vi "ui_Library Query Listed String.vi"(0 "prompt":string, 7 "list of strings":string[](array[string]), 11 "default (persist)":string) -> (4 "OKed?":bool, 8 "selected string":string)   [LabVIEW 2012]
doc: "Allows a string to be easily selected from a list of candidate strings. The prompt explaining what is in need of being selected is shown in the titlebar. It is possible to type in the string, pick it from the list, or type part of the string until the list of candidates is sufficiently reduced to allow quick selection from the list."
uses:
  typedefs/t_Library Query Listed String States.ctl
panel:
  in  "selected":string
  in  "list":i32(listbox)
  in  "cancel":bool
  in  "OK":bool
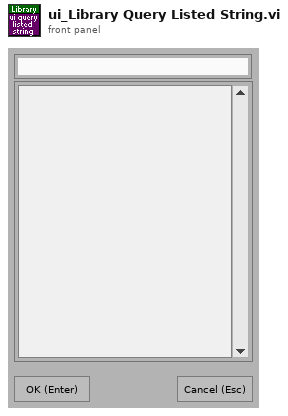
[diagram p1: front panel]
types:
  T1 = typedef "t_Library Query Listed String States.ctl" = enum16{"empty queue", "poll size", "update selected", "filter list", "show list", "OK", "initialize", "init controls", "init check list", "init persist", "init filter", "cleanup", "stop"}
  T2 = typedef "lveventtype.ctl" = enum32{"Null", "Timeout", "Annotation Menu Selection", "Annotation Menu Selection?", "App Instance Close", "App Instance Close?", "Autoscale Range Change", "Cell Edit", "Cell Edit?", "Cursor Grab", "Cursor Grab?", "Cursor Menu Selection", "Cursor Menu Selection?", "Cursor Move", "Cursor Release", "Data Change", "Direction Change", "Display State Change", "Drag Ended", "Drag Enter", "Drag Leave", "Drag Over", "Drag Source Update", "Drag Starting", "Drag Starting?", "Drop", "Exec State Change", "Key Down", "Key Down?", "Key Repeat", "Key Repeat?", "Key Up", "Listbox Double Click", "Menu Activation?", "Menu Selection (App)", "Menu Selection? (App)", "Menu Selection (User)", "Mouse Down", "Mouse Down?", "Mouse Enter", "Mouse Leave", "Mouse Move", "Mouse Up", "NI Security User Change (App)", "Pane Size", "Panel Close", "Panel Close?", "Panel Resize", "Plot Attribute Change", "Scale Range Change", "Shortcut Menu Activation?", "Shortcut Menu Selection (App)", "Shortcut Menu Selection? (App)", "Shortcut Menu Selection (User)", "Tree Double Click", "Tree Drag", "Tree Drag?", "Tree Drop", "Tree Drop?", "Tree Item Close", "Tree Item Close?", "Tree Item Open", "Tree Item Open?", "Value Change"}
  T3 = typedef "eventvkey.ctl" = enum16{"ASCII", "Enter", "Return", "Shift", "Ctrl", "Alt", "Cmd", "Opt", "Caps", "NumLock", "Clear", "Break", "Up", "Down", "Left", "Right", "Insert", "Delete", "Home", "End", "PageUp", "PageDown", "Escape", "Help", "Pause", "ScrollLock", "F1", "F2", "F3", "F4", "F5", "F6", "F7", "F8", "F9", "F10", "F11", "F12", "F13", "F14", "F15", "F16", "F17", "F18", "F19", "F20", "F21", "F22", "F23", "F24", "Play", "VolumeUp", "VolumeDown", "Mute", "Two Byte Char"}
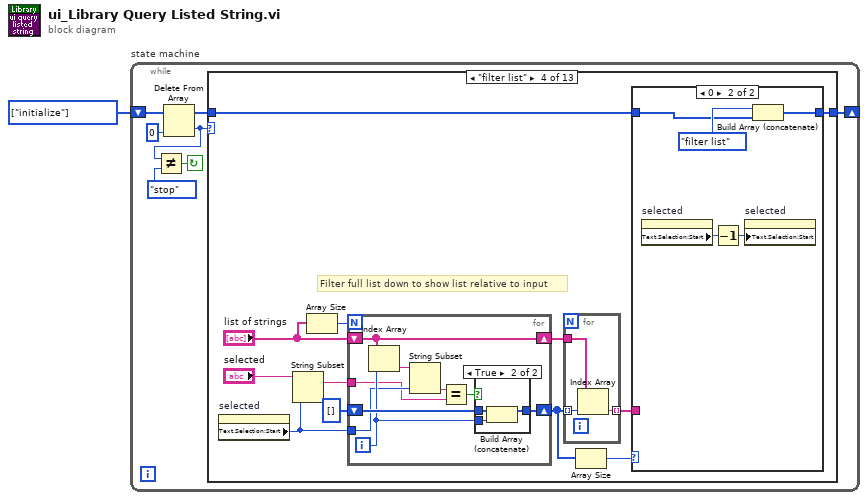
[diagram p0: block diagram]
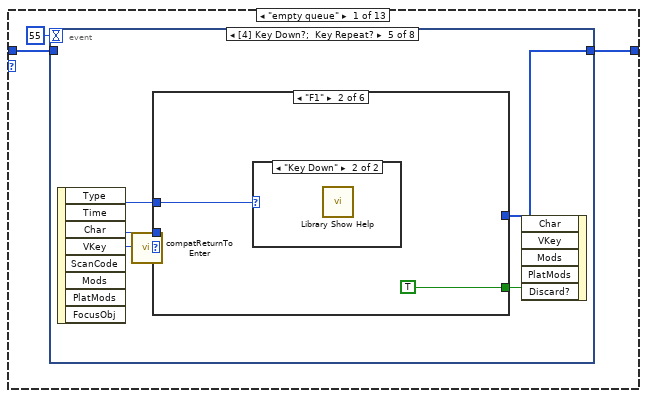
[diagram p2: hidden frame]
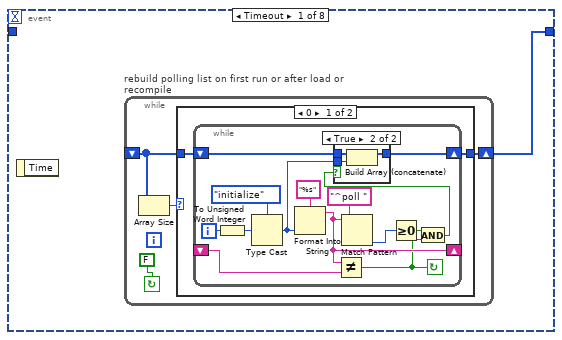
[diagram p3: hidden frame]
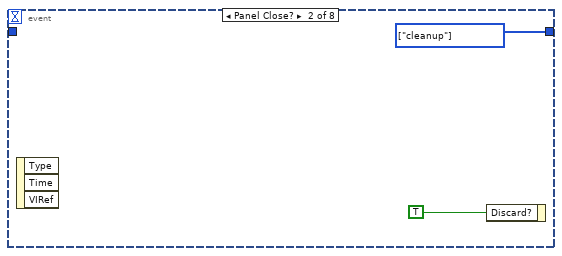
[diagram p6: hidden frame]
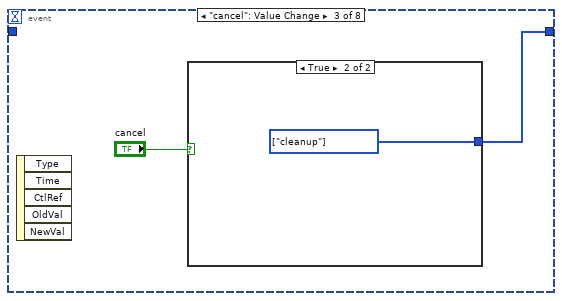
[diagram p7: hidden frame]
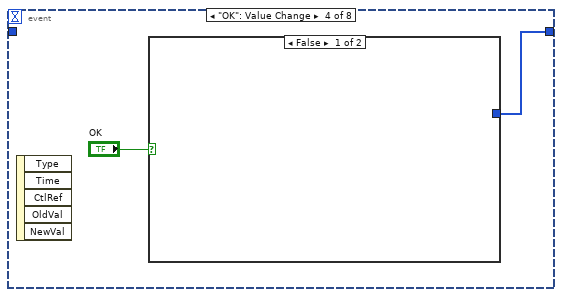
[diagram p9: hidden frame]
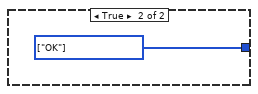
[diagram p10: hidden frame]
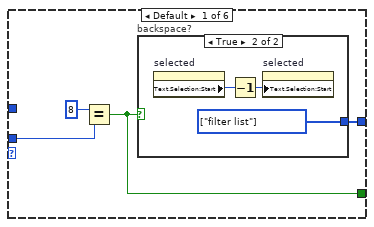
[diagram p11: hidden frame]
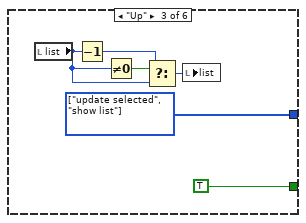
[diagram p14: hidden frame]
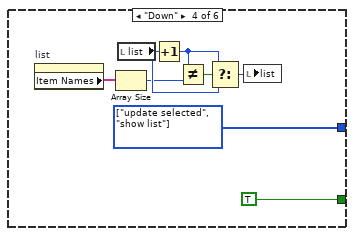
[diagram p15: hidden frame]
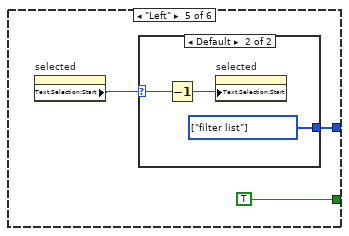
[diagram p16: hidden frame]
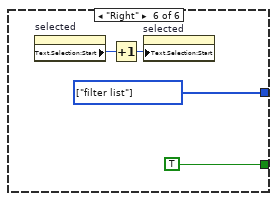
[diagram p18: hidden frame]
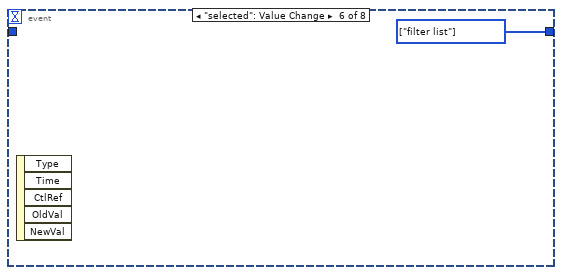
[diagram p19: hidden frame]
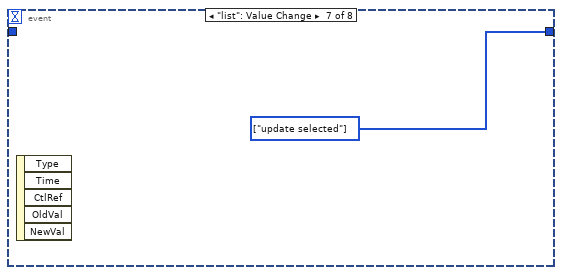
[diagram p20: hidden frame]
diagram:
  w1 = T1[] [enum."initialize"] items=["empty queue", "poll size", "update selected", "filter list", "show list", "OK", "initialize", "init controls", "init check list", "init persist", "init filter", "cleanup", "stop"] ("Array Constant")
  n1 = while "state machine" {
    shift-left: w1 -> [w5]
    shift-right: [w8] -> _
    stop <- w7 continue-if-true
    n2 = Delete From Array(array=w5, index=0) -> (deleted portion=w2:T1, array with subset deleted=w4:T1[])  [unwired: 1 in]
    n3 = Not Equal?(x=w2, y=t_Library_Query_Listed_String_States."stop" ("states")) -> (x != y?=w7:bool)
    n4 = case "Case" shown="\"filter list\"" w2 {
      tunnel: [w11 w91 w108 w119 w146 w180 w182 w212 w214 w220 w230 w234 w235] -> w8
      tunnel: w4 -> [w9 w91 w108 w120 w146 _ _ w212 w215 w220 w231 _ w235]
      frame "empty queue" {
        n5 = event shown="[4] Key Down?;  Key Repeat?" {
          selector: _ -> [_ _ _ _ _ _ _ _]
          dyn-events: _ -> [_ _ _ _ _ _ _ _]
          timeout: 55 -> [_ _ _ _ _ _ _ _]
          tunnel: [w12 w39 w40 w43 w48 w85 w86 w88] -> w11
          tunnel: w9 -> [_ _ _ _ _ _ _ _]
          event Timeout {
            n6 = event-data() -> ()  [unwired: 1 in, 1 out]
            n7 = while "rebuild polling list on first run or after load or recompile" {
              shift-left: _ -> [w15]
              shift-right: [w14] -> w12
              stop <- FALSE continue-if-true
              n8 = Array Size(array=w15) -> (size(s)=w16:i32)
              n9 = case shown="0" w16 {
                tunnel: [w17 w37] -> w14
                tunnel: w15 -> [w18 w37]
                frame 0 {
                  n10 = while {
                    shift-left: w18 -> [w27]
                    shift-right: [w25] -> w17
                    shift-left: _ -> [w29]
                    shift-right: [w24] -> _
                    i -> [w32]
                    stop <- w20 continue-if-true
                    n11 = To Unsigned Word Integer(number=w32) -> (unsigned 16bit integer=w30:u16)
                    n12 = Type Cast(type=t_Library_Query_Listed_String_States."initialize" ("states"), x=w30) -> (*(type *) &x=w26:T1)
                    n13 = Format Into String(format string="%s" ("Format String"), w26) -> (resulting string=w24:string)  [unwired: 2 in, 1 out]
                    n14 = Not Equal?(x=w24, y=w29) -> (x != y?=w20:bool)
                    n15 = Match Pattern(string=w24, regular expression="^poll ") -> (offset past match=w22:i32)  [unwired: 1 in, 3 out]
                    n16 = Greater Or Equal To 0?(x=w22) -> (x >= 0?=w21:bool)
                    n17 = And(x=w21, y=w20) -> (x .and. y?=w19:bool)
                    n18 = case shown="True" w19 {
                      tunnel: w27 -> [w33 w36]
                      tunnel: w26 -> [_ w35]
                      tunnel: [w33 w34] -> w25
                      frame False {
                      }
                      frame True {
                        n19 = Build Array (concatenate)(w36, w35) -> (w34:T1[])
                      }
                    }
                  }
                }
                frame Default {
                }
              }
            }
          }
          event Panel Close? {
            w39 = T1[] [enum."cleanup"] items=["empty queue", "poll size", "update selected", "filter list", "show list", "OK", "initialize", "init controls", "init check list", "init persist", "init filter", "cleanup", "stop"] ("Array Constant")
            n20 = event-data() -> ()  [unwired: 1 in, 3 out]
            n21 = event-data("Discard?"=TRUE) -> ()  [unwired: 1 in, 1 out]
          }
          event "cancel": Value Change {
            n22 = event-data() -> ()  [unwired: 1 in, 5 out]
            n23 = case shown="True" "cancel" {
              tunnel: [_ w42] -> w40
              frame False {
              }
              frame True {
                w42 = T1[] [enum."cleanup"] items=["empty queue", "poll size", "update selected", "filter list", "show list", "OK", "initialize", "init controls", "init check list", "init persist", "init filter", "cleanup", "stop"] ("Array Constant")
              }
            }
          }
          event "OK": Value Change {
            n24 = event-data() -> ()  [unwired: 1 in, 5 out]
            n25 = case shown="False" "OK" {
              tunnel: [_ w45] -> w43
              frame False {
              }
              frame True {
                w45 = T1[] [enum."OK"] items=["empty queue", "poll size", "update selected", "filter list", "show list", "OK", "initialize", "init controls", "init check list", "init persist", "init filter", "cleanup", "stop"] ("Array Constant")
              }
            }
          }
          event Key Down?; event type 5.0.x8000000b {
            n26 = event-data() -> ("Type"=w47:T2, "Char"=w49:i16, "VKey"=w46:T3)  [unwired: 1 in, 5 out]
            n27 = call <vilib>:"compatReturnToEnter.vi"("VKey"=w46) -> ("VKey"=w51:T3)
            n28 = case shown="\"F1\"" w51 {
              tunnel: [w52 TRUE ("Discard?") TRUE ("Discard?") TRUE ("Discard?") TRUE ("Discard?") TRUE ("Discard?")] -> w50
              tunnel: w49 -> [w55 _ _ _ _ _]
              tunnel: [w53 _ w66 w74 w76 w83] -> w48
              tunnel: w47 -> [_ w59 _ _ _ _]
              frame Default {
                n29 = Equal?(x=i16 8, y=w55) -> (x = y?=w52:bool)
                n30 = case "backspace?" shown="True" w52 {
                  tunnel: [_ w58] -> w53
                  frame False {
                  }
                  frame True {
                    w58 = T1[] [enum."filter list"] items=["empty queue", "poll size", "update selected", "filter list", "show list", "OK", "initialize", "init controls", "init check list", "init persist", "init filter", "cleanup", "stop"] ("Array Constant")
                    n31 = property on="selected" class="Str"() -> ("Text.Selection:Start"=w57:u32)  [unwired: 2 in, 2 out]
                    n32 = Decrement(x=w57) -> (x-1=w56:u32)
                    n33 = property on="selected" class="Str"("Text.Selection:Start"=w56) -> ()  [unwired: 2 in, 2 out]
                  }
                }
              }
              frame "F1" {
                n34 = case shown="\"Key Down\"" w59 {
                  frame Default {
                  }
                  frame "Key Down" {
                    n35 = call "Library Show Help.vi"() -> ()  [unwired: 1 in]
                  }
                }
              }
              frame "Up" {
                w66 = T1[] [enum."update selected", enum."show list"] items=["empty queue", "poll size", "update selected", "filter list", "show list", "OK", "initialize", "init controls", "init check list", "init persist", "init filter", "cleanup", "stop"] ("Array Constant")
                n36 = local read "list"() -> (w61:i32)
                n37 = Decrement(x=w61) -> (x-1=w62:i32)
                n38 = Not Equal To 0?(x=w61) -> (x != 0?=w64:bool)
                n39 = Select(t=w62, s=w64, f=w61) -> (s? t:f=w63:i32)
                n40 = local write "list"(w63) -> ()
              }
              frame "Down" {
                w74 = T1[] [enum."update selected", enum."show list"] items=["empty queue", "poll size", "update selected", "filter list", "show list", "OK", "initialize", "init controls", "init check list", "init persist", "init filter", "cleanup", "stop"] ("Array Constant")
                n41 = property on="list" class="LstBox (strict)"() -> ("Item Names"=w67:string[])  [unwired: 2 in, 2 out]
                n42 = Array Size(array=w67) -> (size(s)=w68:i32)
                n43 = local read "list"() -> (w69:i32)
                n44 = Increment(x=w69) -> (x+1=w70:i32)
                n45 = Not Equal?(x=w70, y=w68) -> (x != y?=w72:bool)
                n46 = Select(t=w70, s=w72, f=w69) -> (s? t:f=w71:i32)
                n47 = local write "list"(w71) -> ()
              }
              frame "Left" {
                n48 = property on="selected" class="Str"() -> ("Text.Selection:Start"=w75:u32)  [unwired: 2 in, 2 out]
                n49 = case shown="Default" w75 {
                  selector: w75 -> [_ w78]
                  tunnel: [_ w80] -> w76
                  frame 0 {
                  }
                  frame Default {
                    w80 = T1[] [enum."filter list"] items=["empty queue", "poll size", "update selected", "filter list", "show list", "OK", "initialize", "init controls", "init check list", "init persist", "init filter", "cleanup", "stop"] ("Array Constant")
                    n50 = Decrement(x=w78) -> (x-1=w79:u32)
                    n51 = property on="selected" class="Str"("Text.Selection:Start"=w79) -> ()  [unwired: 2 in, 2 out]
                  }
                }
              }
              frame "Right" {
                w83 = T1[] [enum."filter list"] items=["empty queue", "poll size", "update selected", "filter list", "show list", "OK", "initialize", "init controls", "init check list", "init persist", "init filter", "cleanup", "stop"] ("Array Constant")
                n52 = property on="selected" class="Str"() -> ("Text.Selection:Start"=w82:u32)  [unwired: 2 in, 2 out]
                n53 = Increment(x=w82) -> (x+1=w81:u32)
                n54 = property on="selected" class="Str"("Text.Selection:Start"=w81) -> ()  [unwired: 2 in, 2 out]
              }
            }
            n55 = event-data("Discard?"=w50) -> ()  [unwired: 5 in, 1 out]
          }
          event "selected": Value Change {
            w85 = T1[] [enum."filter list"] items=["empty queue", "poll size", "update selected", "filter list", "show list", "OK", "initialize", "init controls", "init check list", "init persist", "init filter", "cleanup", "stop"] ("Array Constant")
            n56 = event-data() -> ()  [unwired: 1 in, 5 out]
          }
          event "list": Value Change {
            w86 = T1[] [enum."update selected"] items=["empty queue", "poll size", "update selected", "filter list", "show list", "OK", "initialize", "init controls", "init check list", "init persist", "init filter", "cleanup", "stop"] ("Array Constant")
            n57 = event-data() -> ()  [unwired: 1 in, 5 out]
          }
          event Mouse Up {
            n58 = event-data() -> ()  [unwired: 1 in, 7 out]
            n59 = property on="list" class="LstBox (strict)"() -> ("Double-Click"=w87:i32)  [unwired: 2 in, 2 out]
            n60 = case shown="Default" w87 {
              tunnel: [_ w90] -> w88
              frame -1 {
                n61 = property on="selected" class="Str"("Key Focus"=TRUE) -> ()  [unwired: 2 in, 2 out]
              }
              frame Default {
                w90 = T1[] [enum."OK"] items=["empty queue", "poll size", "update selected", "filter list", "show list", "OK", "initialize", "init controls", "init check list", "init persist", "init filter", "cleanup", "stop"] ("Array Constant")
              }
            }
          }
        }
      }
      frame "poll size" {
        w93 = u32 9  # To match the size of the listbox...
        n62 = property on="list" class="LstBox (strict)"() -> ("Bounds:Width"=w92:u32)  [unwired: 2 in, 2 out]
        n63 = property on="selected" class="Str"() -> ("Text Size:Width"=w97:u32, "Key Focus"=w95:bool)  [unwired: 2 in, 2 out]
        n64 = Subtract(x=w92, y=w93) -> (x-y=w94:u32)
        n65 = Not Equal?(x=w94, y=w97) -> (x != y?=w96:bool)
        n66 = case shown="True" w96 {
          tunnel: w94 -> [_ w99]
          tunnel: w95 -> [_ w98]
          frame False {
          }
          frame True {
            n67 = stacked-sequence {
              tunnel: w99 -> [w101 _]
              tunnel: w98 -> [_ w102]
              frame #0 {
                n68 = property on="selected" class="Str"("Key Focus"=FALSE, "Text Size:Width"=w101) -> ()  [unwired: 2 in, 2 out]
              }
              frame #1 {
                n69 = property on="selected" class="Str"("Key Focus"=w102) -> ()  [unwired: 2 in, 2 out]
              }
            }
          }
        }
      }
      frame "update selected" {
        n70 = property on="list" class="LstBox (strict)"() -> ("Item Names"=w104:string[])  [unwired: 2 in, 2 out]
        n71 = Index Array(array=w104, index="list") -> (element=w105:string)
        n72 = String Length(string=w105) -> (length=w107:i32)
        n73 = To Unsigned Long Integer(number=w107) -> (unsigned 32bit integer=w106:u32)
        n74 = property on="selected" class="Str"("Value"=w105, "Text.Selection:End"=w106) -> ()  [unwired: 2 in, 2 out]
      }
      frame "filter list" {
        # "Filter full list down to show list relative to input"
        n75 = property on="selected" class="Str"() -> ("Text.Selection:Start"=w116:u32)  [unwired: 2 in, 2 out]
        n76 = String Subset(string="selected", length (rest)=w116) -> (substring=w114:string)  [unwired: 1 in]
        n77 = Array Size(array="list of strings") -> (size(s)=w115:i32)
        n78 = for {
          N: w115 -> [_]
          shift-right: [w133] -> w111
          shift-left: i32[] [] -> [w141]
          tunnel: w114 -> [w136]
          shift-right: [w139] -> w112
          shift-left: "list of strings" -> [w139]
          tunnel: w116 -> [w138]
          i -> [w140]
          n79 = Index Array(array=w139, index=w140) -> (element=w137:string)
          n80 = String Subset(string=w137, length (rest)=w138) -> (substring=w134:string)  [unwired: 1 in]
          n81 = Equal?(x=w134, y=w136) -> (x = y?=w135:bool)
          n82 = case shown="True" w135 {
            tunnel: w141 -> [w142 w145]
            tunnel: [w142 w144] -> w133
            tunnel: w140 -> [_ w143]
            frame False {
            }
            frame True {
              n83 = Build Array (concatenate)(w145, w143) -> (w144:i32[])
            }
          }
        }
        n84 = for {
          tunnel: w111 -> [w132] mode=indexing
          tunnel: [w131] -> w109 mode=indexing
          tunnel: w112 -> [w130]
          n85 = Index Array(array=w130, index=w132) -> (element=w131:string)
        }
        n86 = Array Size(array=w111) -> (size(s)=w110:i32)
        n87 = case shown="0" w110 {
          tunnel: w120 -> [w124 w125]
          tunnel: [w123 w126] -> w119
          tunnel: w109 -> [w121 _]
          frame Default {
            n88 = property on="list" class="LstBox (strict)"("Item Names"=w121) -> ()  [unwired: 2 in, 2 out]
            n89 = Build Array (concatenate)(t_Library_Query_Listed_String_States."show list" ("states"), w124) -> (w123:T1[])
          }
          frame 0 {
            n90 = property on="selected" class="Str"() -> ("Text.Selection:Start"=w128:u32)  [unwired: 2 in, 2 out]
            n91 = Decrement(x=w128) -> (x-1=w129:u32)
            n92 = property on="selected" class="Str"("Text.Selection:Start"=w129) -> ()  [unwired: 2 in, 2 out]
            n93 = Build Array (concatenate)(t_Library_Query_Listed_String_States."filter list" ("states"), w125) -> (w126:T1[])
          }
        }
      }
      frame "show list" {
        n94 = property on="list" class="LstBox (strict)"() -> ("Item Names"=w152:string[])  [unwired: 2 in, 2 out]
        n95 = local read "selected"() -> (w153:string)
        n96 = Array Size(array=w152) -> (size(s)=w157:i32)
        n97 = property on="list" class="LstBox (strict)"() -> ("Number of Rows"=w160:u32, "Top Row"=w158:i32)  [unwired: 2 in, 2 out]
        n98 = Decrement(x=w157) -> (x-1=w154:i32)
        n99 = Search 1D Array(1D array=w152, element=w153) -> (index of element=w151:i32)  [unwired: 1 in]
        n100 = Greater Than 0?(x=w151) -> (x > 0?=w150:bool)
        n101 = Add(x=w160, y=w158) -> (x+y=w159:u32)
        n102 = Select(t=w151, s=w150, f=0) -> (s? t:f=w148:i32)
        n103 = property on="selected" class="Str"("Key Focus"=TRUE) -> ()  [unwired: 2 in, 2 out]
        n104 = In Range and Coerce(upper limit=w159, x=w148, lower limit=w158) -> (In Range?=w161:bool)  [unwired: 1 out]
        n105 = local write "list"(w148) -> ()
        n106 = case shown="True" w161 {
          tunnel: w148 -> [w167 _]
          tunnel: w159 -> [w169 _]
          tunnel: w160 -> [w165 _]
          tunnel: w154 -> [_ w175]
          tunnel: w160 -> [_ w174]
          tunnel: w158 -> [_ w171]
          frame False {
            n107 = Subtract(x=w167, y=w165) -> (x-y=w166:u32)
            n108 = Less?(x=w167, y=w169) -> (x < y?=w168:bool)
            n109 = Increment(x=w166) -> (x+1=w164:u32)
            n110 = Select(t=w167, s=w168, f=w164) -> (s? t:f=w163:u32)
            n111 = property on="list" class="LstBox (strict)"("Top Row"=w163) -> ()  [unwired: 2 in, 2 out]
          }
          frame True {
            n112 = Less?(x=w175, y=w174) -> (x < y?=w173:bool)
            n113 = Select(t=0 ("upper limit"), s=w173, f=w171) -> (s? t:f=w170:i32)
            n114 = property on="list" class="LstBox (strict)"("Top Row"=w170) -> ()  [unwired: 2 in, 2 out]
          }
        }
        n115 = Index Array(array=w152, index=w148) -> (element=w147:string)
        n116 = String Length(string=w147) -> (length=w156:i32)
        n117 = To Unsigned Long Integer(number=w156) -> (unsigned 32bit integer=w155:u32)
        n118 = property on="selected" class="Str"("Value"=w147, "Text.Selection:End"=w155) -> ()  [unwired: 2 in, 2 out]
      }
      frame "OK" {
        w180 = T1[] [enum."cleanup"] items=["empty queue", "poll size", "update selected", "filter list", "show list", "OK", "initialize", "init controls", "init check list", "init persist", "init filter", "cleanup", "stop"] ("Array Constant")
        n119 = property on="list" class="LstBox (strict)"() -> ("Item Names"=w181:string[])  [unwired: 2 in, 2 out]
        n120 = local read "list"() -> (w177:i32)
        n121 = Index Array(array=w181, index=w177) -> (element=w176:string)
        "selected string" <- w176
        n122 = Empty String/Path?(string/path=w176) -> (empty?=w179:bool)
        n123 = Not(x=w179) -> (.not. x?=→"OKed?":bool)
      }
      frame "initialize" {
        n124 = while "rebuild init list on first run or after load or recompile" {
          shift-left: _ -> [w185]
          shift-right: [w184] -> w182
          stop <- FALSE continue-if-true
          n125 = Array Size(array=w185) -> (size(s)=w186:i32)
          n126 = case shown="0" w186 {
            tunnel: [w187 w207] -> w184
            tunnel: w185 -> [w188 w207]
            frame 0 {
              n127 = while {
                shift-left: w188 -> [w197]
                shift-right: [w195] -> w187
                shift-left: _ -> [w199]
                shift-right: [w194] -> _
                i -> [w202]
                stop <- w190 continue-if-true
                n128 = To Unsigned Word Integer(number=w202) -> (unsigned 16bit integer=w200:u16)
                n129 = Type Cast(type=t_Library_Query_Listed_String_States."initialize" ("states"), x=w200) -> (*(type *) &x=w196:T1)
                n130 = Format Into String(format string="%s" ("Format String"), w196) -> (resulting string=w194:string)  [unwired: 2 in, 1 out]
                n131 = Not Equal?(x=w194, y=w199) -> (x != y?=w190:bool)
                n132 = Match Pattern(string=w194, regular expression="^init ") -> (offset past match=w192:i32)  [unwired: 1 in, 3 out]
                n133 = Greater Or Equal To 0?(x=w192) -> (x >= 0?=w191:bool)
                n134 = And(x=w191, y=w190) -> (x .and. y?=w189:bool)
                n135 = case shown="True" w189 {
                  tunnel: w197 -> [w203 w206]
                  tunnel: w196 -> [_ w205]
                  tunnel: [w203 w204] -> w195
                  frame False {
                  }
                  frame True {
                    n136 = Build Array (concatenate)(w206, w205) -> (w204:T1[])
                  }
                }
              }
            }
            frame Default {
            }
          }
        }
      }
      frame "init controls" {
        n137 = local write "selected string"("") -> ()
        n138 = local write "OKed?"(FALSE ("OKed?")) -> ()
        n139 = property on="selected" class="Str"("Key Focus"=TRUE) -> ()  [unwired: 2 in, 2 out]
        n140 = local write "list"(0 ("tag list")) -> ()
        n141 = property class="VI"("Front Panel Window:Title"="prompt") -> ()  [unwired: 2 in, 2 out]
      }
      frame "init check list" {
        w216 = T1[] [enum."stop"] items=["empty queue", "poll size", "update selected", "filter list", "show list", "OK", "initialize", "init controls", "init check list", "init persist", "init filter", "cleanup", "stop"] ("Array Constant")
        n142 = local read "list of strings"() -> (w219:string[])
        n143 = Array Size(array=w219) -> (size(s)=w218:i32)
        n144 = Not Equal To 0?(x=w218) -> (x != 0?=w217:bool)
        n145 = Select(t=w215, s=w217, f=w216) -> (s? t:f=w214:T1[])
      }
      frame "init persist" {
        n146 = flat-sequence {
          frame #0 {
            n147 = call "Libary Persist Position and Controls.vi"("action"=enum16{"save", "load"}."load") -> ()  [unwired: 13 in, 2 out]
          }
          frame #1 {
            n148 = Empty String/Path?(string/path="default (persist)") -> (empty?=w223:bool)
            n149 = case shown="False" w223 {
              tunnel: "default (persist)" -> [w224 _]
              frame False {
                n150 = local write "selected"(w224) -> ()
              }
              frame True {
              }
            }
          }
        }
      }
      frame "init filter" {
        n151 = local read "selected"() -> (w228:string)
        n152 = String Length(string=w228) -> (length=w227:i32)
        n153 = To Unsigned Long Integer(number=w227) -> (unsigned 32bit integer=w226:u32)
        n154 = property on="selected" class="Str"("Text.Selection:Start"=u32 0, "Text.Selection:End"=w226) -> ()  [unwired: 2 in, 2 out]
        n155 = Build Array (concatenate)(t_Library_Query_Listed_String_States."filter list" ("states"), w231) -> (w230:T1[])
      }
      frame "cleanup" {
        w234 = T1[] [enum."stop"] items=["empty queue", "poll size", "update selected", "filter list", "show list", "OK", "initialize", "init controls", "init check list", "init persist", "init filter", "cleanup", "stop"] ("Array Constant")
        n156 = property on="list" class="LstBox (strict)"("Item Names"=string[] []) -> ()  [unwired: 2 in, 2 out]
        n157 = call "Libary Persist Position and Controls.vi"("action"=enum16{"save", "load"}."save") -> ()  [unwired: 13 in, 2 out]
      }
      frame "stop" {
        n158 = invoke class="VI" method="FP.Close"() -> ()  [unwired: 3 in, 3 out]
      }
    }
  }
